vi "get extio settings.vi"(8 "error in (no error)":errorcluster, 10 "extio_settings":T1, 11 "id":i32) -> (0 "error out":errorcluster, 2 "extio_settings out":T1, 3 "function return":i32)   [LabVIEW 2012, in "libximc.lvlib"]
doc: "result_t XIMC_API get_extio_settings (device_t id, extio_settings_t* extio_settings);"
uses:
  libximc.lvlib
  libximc.dll
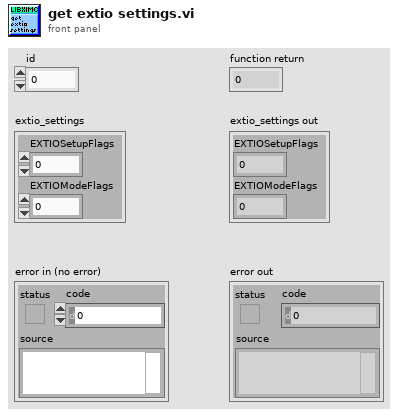
[diagram p1: front panel]
types:
  T1 = cluster{"EXTIOSetupFlags":u32, "EXTIOModeFlags":u32}
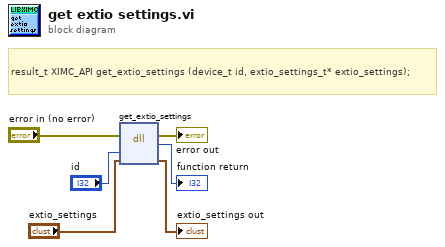
[diagram p0: block diagram]
diagram:
  # "result_t XIMC_API get_extio_settings (device_t id, extio_settings_t* extio_settings);"
  n1 = dll-call lib="C:/Users/Stepan/Downloads/labview_2.9.11_testgen_thread/libximc.*" fn="get_extio_settings"(error in="error in (no error)", "id"="id", "extio_settings"="extio_settings") -> (error out=→"error out":errorcluster, →"function return":i32, "extio_settings"=→"extio_settings out":T1)  [unwired: 3 in, 1 out]
